vi "Create One Frame Script.vi"(8 "error in (no error)":errorcluster, 10 "Config String":string, 11 "BML_LS Pattern Creator in":refnum<class "BML_LS Pattern Creator.lvclass">) -> (0 "error out":errorcluster, 1 "Pattern Name out":string, 2 "Script out":string, 3 "BML_LS Pattern Creator out":refnum<class "BML_LS Pattern Creator.lvclass">)   [LabVIEW 2018, in "BML_LS Pattern Creator.lvlib" / "BML_LS Pattern Creator.lvclass"]
uses:
  BML_LS Pattern Creator.lvclass
  C:/P4 Workspace/PC Client/Solutions/5g_eap/trunk/1.0/HiSi5GmmWave/Pattern_Gen_Tool/Plugins/Protocols/BML Pattern Creater.lvlibp/Plugins/SouceCode/BML Pattern Creater/BML Pattern Creater.lvclass
  C:/P4 Workspace/PC Client/Solutions/5g_eap/trunk/1.0/HiSi5GmmWave/Pattern_Gen_Tool/Interfaces/Protocol Interface.lvlibp/Interfaces/Protocol Interface/Protocol Interface.lvclass
  Protocols/BML Pattern Creater.lvlibp/Plugins/SouceCode/BML Pattern Creater/Special Frame.ctl
  Protocols/BML Pattern Creater.lvlibp/Plugins/SouceCode/BML Pattern Creater/Read R_W_.vi
  Protocols/BML Pattern Creater.lvlibp/Plugins/SouceCode/BML Pattern Creater/Read Pattern_Name.vi
  Interfaces/Protocol Interface.lvlibp/Interfaces/Protocol Interface/Read Num of cycle Rd.vi
  Protocols/BML Pattern Creater.lvlibp/Plugins/SouceCode/BML Pattern Creater/BML Pattern Creater.lvclass
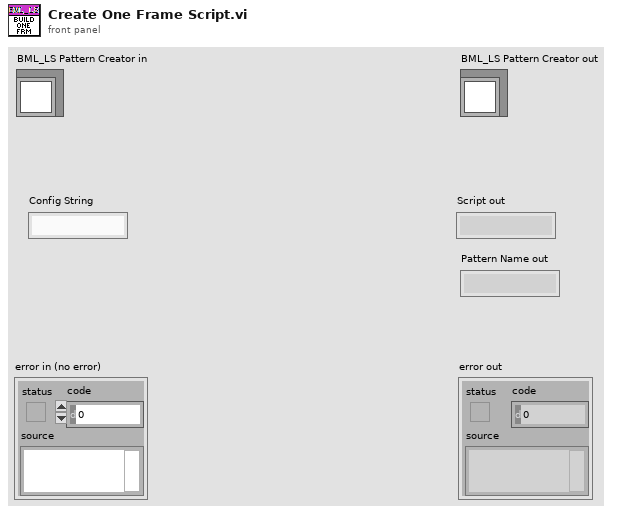
[diagram p1: front panel]
types:
  T1 = typedef "BML Pattern Creater.lvlibp/BML Pattern Creater.lvclass/Special Frame.ctl" = enum16{"Sync Header", "BML Header", "SW Trig", "SetID State", "Exit SetID State", "SW Reset", "Wait"}
  T2 = typedef "BML Pattern Creater.lvlibp/RW Options.ctl" = enum16{"Read", "Write", "R/W"}
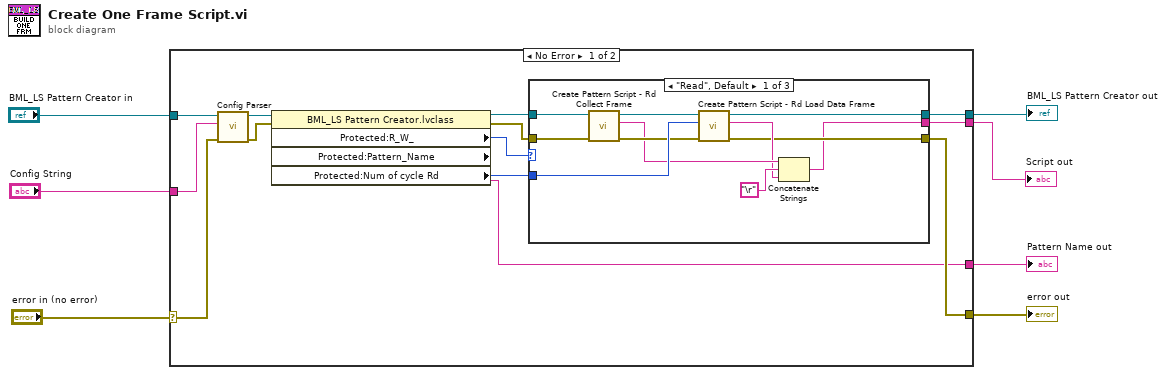
[diagram p0: block diagram]
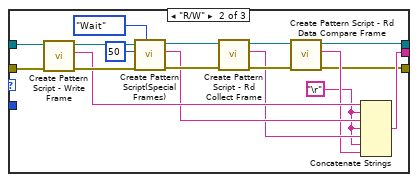
[diagram p2: hidden frame]
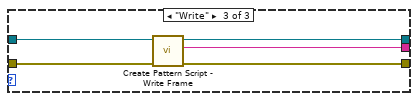
[diagram p3: hidden frame]
diagram:
  n1 = case shown="No Error" "error in (no error)" {
    selector: "error in (no error)" -> [w18 w55]
    tunnel: "BML_LS Pattern Creator in" -> [w20 w56]
    tunnel: "Config String" -> [w19 _]
    tunnel: [w12 w56] -> w4
    tunnel: [w11 _] -> w3
    tunnel: [w10 w55] -> w2
    tunnel: [w9 _] -> w1
    frame No Error {
      n2 = call "Config Parser.vi"("error in (no error)"=w18, "Config String"=w19, "BML Pattern Creater in"=w20) -> ("error out"=w16:errorcluster, "BML Pattern Creater out"=w17:refnum<class "BML_LS Pattern Creator.lvclass">)  [unwired: 7 in]
      n3 = property class="BML_LS Pattern Creator.lvclass"(reference=w17, error in=w16) -> (reference out=w15:refnum<class "BML_LS Pattern Creator.lvclass">, error out=w13:errorcluster, "Protected:R_W_"=w14:T2, "Protected:Pattern_Name"=w9:string, "Protected:Num of cycle Rd"=w8:u32)
      n4 = case shown="\"Read\", Default" w14 {
        tunnel: w15 -> [w31 w49 w54]
        tunnel: w13 -> [w30 w48 w53]
        tunnel: [w26 w32 w52] -> w12
        tunnel: [w21 w34 w51] -> w11
        tunnel: [w22 w33 w50] -> w10
        tunnel: w8 -> [w29 _ _]
        frame "Read", Default {
          n5 = call "Create Pattern Script - Rd Collect Frame.vi"("error in (no error)"=w30, "BML Pattern Creater.lvclass"=w31) -> ("error out"=w28:errorcluster, "Rd Collect out"=w25:string, "BML Pattern Creater.lvclass"=w27:refnum<class "BML_LS Pattern Creator.lvclass">)  [unwired: 7 in]
          n6 = call "Create Pattern Script - Rd Load Data Frame.vi"("error in (no error)"=w28, "Num of Cycles"=w29, "BML Pattern Creater in"=w27) -> ("error out"=w22:errorcluster, "Rd Capture"=w23:string, "BML Pattern Creater out"=w26:refnum<class "BML_LS Pattern Creator.lvclass">)  [unwired: 6 in]
          n7 = Concatenate Strings(w25, "\r", w23) -> (w21:string)
        }
        frame "R/W" {
          w35 = "\r"
          n8 = call "Create Pattern Script - Write Frame.vi"("error in (no error)"=w48, "BML Pattern Creater in"=w49) -> ("error out"=w47:errorcluster, "Script out"=w39:string, "BML Pattern Creater out"=w46:refnum<class "BML_LS Pattern Creator.lvclass">)  [unwired: 7 in]
          n9 = call "Create Pattern Script(Special Frames).vi"("Special Frame Type"=Special_Frame."Wait", "error in (no error)"=w47, "Num of Timeset"=u32 50, "BML Pattern Creater in"=w46) -> ("error out"=w42:errorcluster, "string out"=w38:string, "BML Pattern Creater out"=w43:refnum<class "BML_LS Pattern Creator.lvclass">)  [unwired: 5 in]
          n10 = call "Create Pattern Script - Rd Collect Frame.vi"("error in (no error)"=w42, "BML Pattern Creater.lvclass"=w43) -> ("error out"=w40:errorcluster, "Rd Collect out"=w37:string, "BML Pattern Creater.lvclass"=w41:refnum<class "BML_LS Pattern Creator.lvclass">)  [unwired: 7 in]
          n11 = call "Create Pattern Script - Rd Data Compare Frame.vi"("error in (no error)"=w40, "BML Pattern Creater in"=w41) -> ("error out"=w33:errorcluster, "RdDataCompare"=w36:string, "BML Pattern Creater out"=w32:refnum<class "BML_LS Pattern Creator.lvclass">)  [unwired: 7 in]
          n12 = Concatenate Strings(w39, w35, w38, w35, w37, w35, w36) -> (w34:string)
        }
        frame "Write" {
          n13 = call "Create Pattern Script - Write Frame.vi"("error in (no error)"=w53, "BML Pattern Creater in"=w54) -> ("error out"=w50:errorcluster, "Script out"=w51:string, "BML Pattern Creater out"=w52:refnum<class "BML_LS Pattern Creator.lvclass">)  [unwired: 7 in]
        }
      }
    }
    frame Error {
    }
  }
  "error out" <- w2
  "BML_LS Pattern Creator out" <- w4
  "Script out" <- w3
  "Pattern Name out" <- w1
